vi "Cargo Test.vi"(10 "Run":bool) -> ()   [LabVIEW 2018]
uses:
  SubSystems/Cargo Intake/Cargo Intake Global.vi
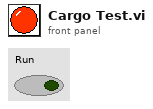
[diagram p1: front panel]
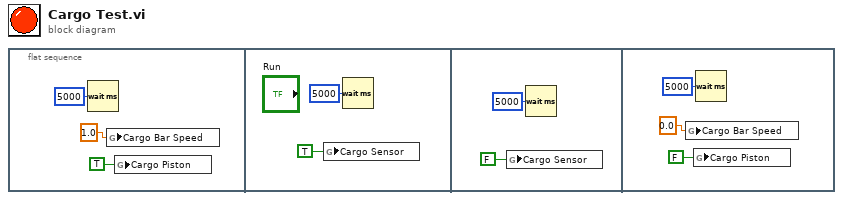
[diagram p0: block diagram]
diagram:
  n1 = flat-sequence {
    frame #0 {
      n2 = Wait (ms)(milliseconds to wait=u32 5000) -> ()  [unwired: 1 out]
      n3 = global write "Cargo Intake Global.vi" "Cargo Bar Speed"(1.0 ("Cargo Bar Speed")) -> ()
      n4 = global write "Cargo Intake Global.vi" "Cargo Piston"(TRUE) -> ()
    }
    frame #1 {
      n5 = global write "Cargo Intake Global.vi" "Cargo Sensor"(TRUE) -> ()
      n6 = Wait (ms)(milliseconds to wait=u32 5000) -> ()  [unwired: 1 out]
    }
    frame #2 {
      n7 = global write "Cargo Intake Global.vi" "Cargo Sensor"(FALSE) -> ()
      n8 = Wait (ms)(milliseconds to wait=u32 5000) -> ()  [unwired: 1 out]
    }
    frame #3 {
      n9 = global write "Cargo Intake Global.vi" "Cargo Bar Speed"(0.0 ("Cargo Bar Speed")) -> ()
      n10 = global write "Cargo Intake Global.vi" "Cargo Piston"(FALSE) -> ()
      n11 = Wait (ms)(milliseconds to wait=u32 5000) -> ()  [unwired: 1 out]
    }
  }
